vi "Joystick Control.vi"(7 "control_request":string, 11 "control_devices_reference":T2) -> (0 "indicatror_joystick_axes":T3, 1 "indicator_joystick_buttons":T5, 2 "indicator_joystick_status":bool, 3 "indicator_joystick_event_reference":refnum<event-registration>, 5 "indicator_joystick_reference":T1)   [LabVIEW 2020]
uses:
  <vilib>/MakerHub/PS4-Controller/Private/Type Defs/PS4 Controller Ref.ctl
  <vilib>/MakerHub/PS4-Controller/Private/Type Defs/Buttons.ctl
  <vilib>/MakerHub/PS4-Controller/Private/Type Defs/Axis.ctl
  <vilib>/MakerHub/PS4-Controller/Private/Type Defs/Indicators/DPad Enum.ctl
  C:/Users/Public/Documents/Photometrics/PMQI-LabViewSamples/Examples/2018/Dependencies/PVCamNET.dll
  Public/Documents/Photometrics/PMQI-LabViewSamples/Examples/2018/Dependencies/PVCamNET.dll
  <vilib>/SmarAct/SmarActCTL/SA_CTL.lvclass
  <vilib>/MakerHub/PS4-Controller/Public/Open First Controller.vi
  <vilib>/MakerHub/PS4-Controller/LMH-PS4.lvlib
panel:
  out "Error Out":errorcluster
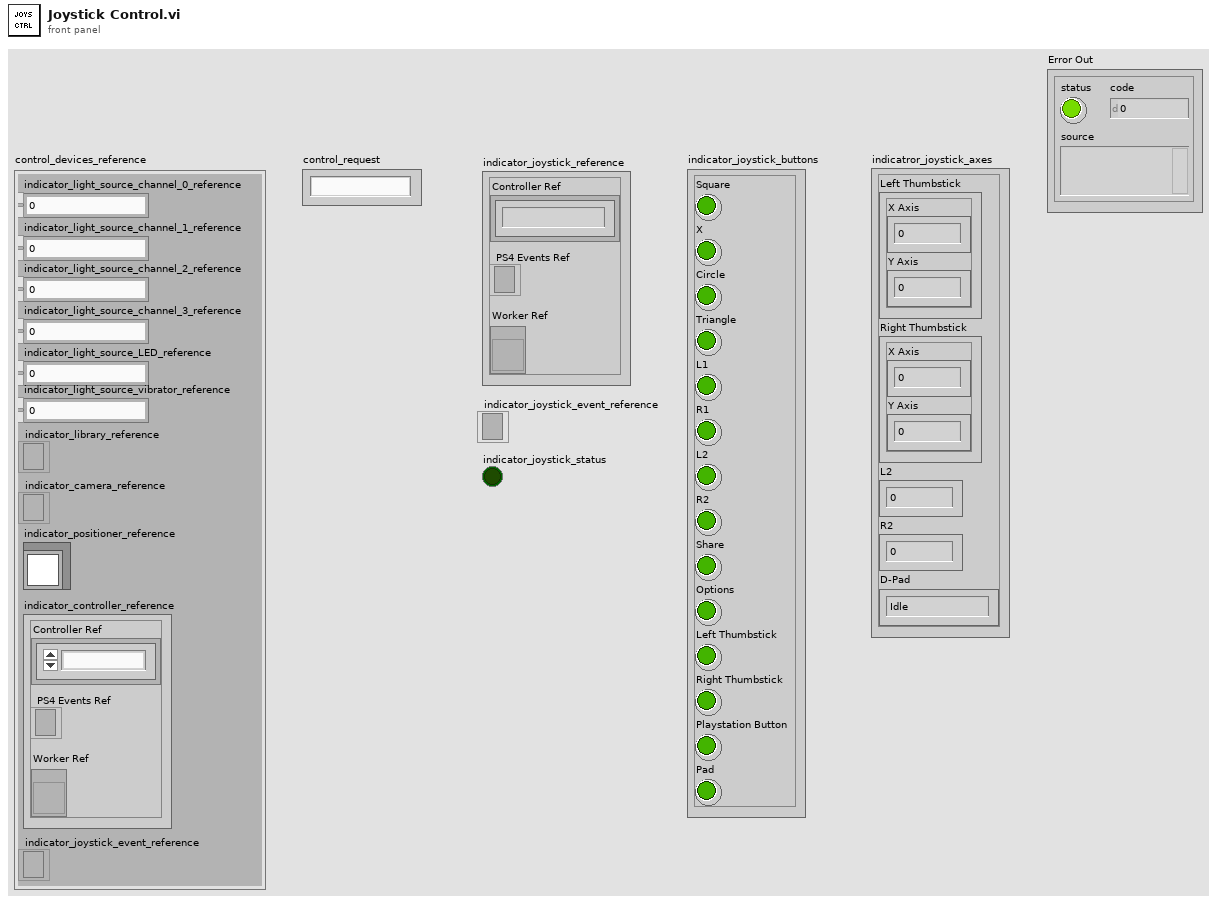
[diagram p1: front panel]
types:
  T1 = typedef "LMH-PS4.lvlib/PS4 Controller Ref.ctl" = cluster{"Controller Ref":refnum<k1>, "PS4 Events Ref":refnum<event-registration>, "Worker Ref":refnum<vi>}
  T2 = cluster{"indicator_light_source_channel_0_reference":u64, "indicator_light_source_channel_1_reference":u64, "indicator_light_source_channel_2_reference":u64, "indicator_light_source_channel_3_reference":u64, "indicator_library_reference":refnum<k24>, "indicator_camera_reference":refnum<k24>, "indicator_positioner_reference":refnum<class "SA_CTL.lvclass">, "indicator_controller_reference":T1, "indicator_joystick_event_reference":refnum<event-registration>, "indicator_light_source_LED_reference":u64, "indicator_light_source_vibrator_reference":u64}
  T3 = typedef "LMH-PS4.lvlib/Axis.ctl" = cluster{"Left Thumbstick":cluster{"X Axis":i32, "Y Axis":i32}, "Right Thumbstick":cluster{"X Axis":i32, "Y Axis":i32}, "L2":i32, "R2":i32, "D-Pad":T4}
  T4 = typedef "LMH-PS4.lvlib/DPad Enum.ctl" = enum16{"Idle", "Up", "Up / Right", "Right", "Down / Right", "Down", "Down / Left", "Left", "Up / Left"}
  T5 = typedef "LMH-PS4.lvlib/Buttons.ctl" = cluster{"Square":bool, "X":bool, "Circle":bool, "Triangle":bool, "L1":bool, "R1":bool, "L2":bool, "R2":bool, "Share":bool, "Options":bool, "Left Thumbstick":bool, "Right Thumbstick":bool, "Playstation Button":bool, "Pad":bool}
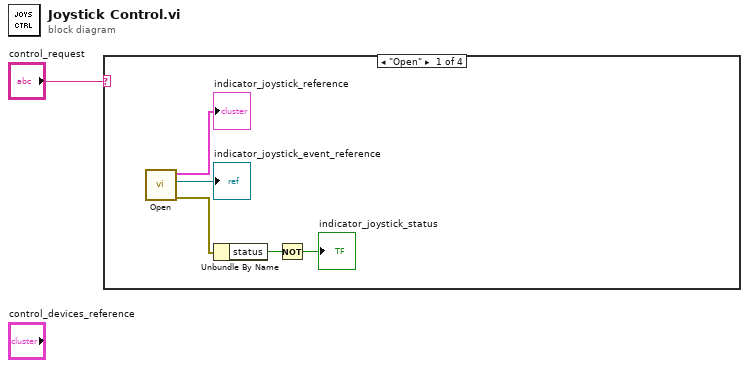
[diagram p0: block diagram]
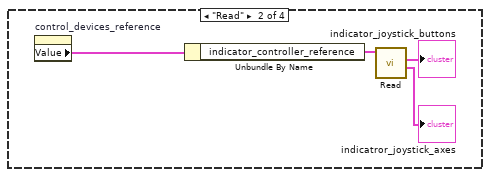
[diagram p2: hidden frame]
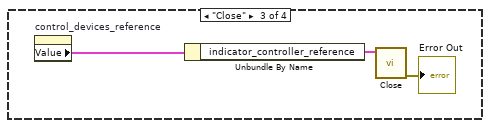
[diagram p3: hidden frame]
diagram:
  n1 = case shown="\"Open\"" "control_request" {
    frame "Open" {
      n2 = call-poly <vilib>:"Open.vi"() -> ("Error Out"=w4:errorcluster, "Event Registration Refnum"=→"indicator_joystick_event_reference":refnum<event-registration>, "PS4 Controller Ref"=→"indicator_joystick_reference":T1)  [unwired: 9 in]
      n3 = Unbundle By Name(w4) -> ("status"=w3:bool)
      n4 = Not(x=w3) -> (.not. x?=→"indicator_joystick_status":bool)
    }
    frame "Read" {
      n5 = property on="control_devices_reference" class="Clust (strict)"() -> ("Value"=w7:T2)  [unwired: 2 in, 2 out]
      n6 = Unbundle By Name(w7) -> ("indicator_controller_reference"=w8:T1)
      n7 = call <vilib>:"Read.vi"("PS4 Controller Ref"=w8) -> ("All Axis"=→"indicatror_joystick_axes":T3, "Buttons"=→"indicator_joystick_buttons":T5)  [unwired: 7 in, 2 out]
    }
    frame "Close" {
      n8 = property on="control_devices_reference" class="Clust (strict)"() -> ("Value"=w13:T2)  [unwired: 2 in, 2 out]
      n9 = Unbundle By Name(w13) -> ("indicator_controller_reference"=w12:T1)
      n10 = call <vilib>:"Close.vi"("PS4 Controller Ref"=w12) -> ("Error Out"=→"Error Out":errorcluster)  [unwired: 10 in]
    }
    frame "Default", Default {
    }
  }
